vi "MiPS_set.vi"(5 "Target Current":dbl, 6 "stop":bool, 7 "Ramp Rate (A/min)":dbl, 8 "error in":errorcluster, 9 "ISOBUS address":T5, 11 "ref_in":T1) -> (0 "error out":errorcluster, 1 "PSU Act Stat":T4, 3 "ref_out":T1, 4 "iPS_msg":string caption="Msg.")   [LabVIEW 2019]
uses:
  Mercury iXX Modules/Public/Controls/ISOBus Address.ctl
  Mercury iXX Modules/Public/Libraries/Magnet/Controls/PSU Actions.ctl
  Mercury iXX Modules/Public/Controls/Mercury Reference.ctl
  Mercury iXX Modules/Public/Controls/Comms Transport Layer.ctl
  Mercury iXX Modules/Private/Controls/Query Dynamic Reference.ctl
  Mercury iXX Modules/Public/Libraries/Magnet/Signals/Set/Target Current (Set).vi
  Mercury iXX Modules/Public/Libraries/Magnet/Signals/Set/Target Current Rate (Set).vi
  Mercury iXX Modules/Public/Libraries/Magnet/Configuration/Set/PSU Action Status (Set).vi
  Mercury iXX Modules/Public/Libraries/Magnet/Configuration/Read/PSU Action Status (Read).vi
  Mercury iXX Modules/Mercury iXX.lvlib
  Mercury iXX Modules/Public/Libraries/Magnet.lvlib
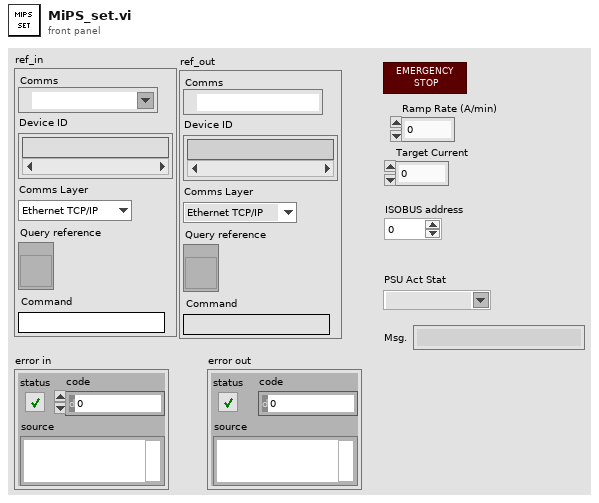
[diagram p1: front panel]
types:
  T1 = typedef "Mercury iXX.lvlib/Mercury Reference.ctl" = cluster{"Comms":refnum<visa-resource-name>, "Device ID":string[], "Comms Layer":T2, "Command":string, "Query reference":T3}
  T2 = typedef "Mercury iXX.lvlib/Comms Transport Layer.ctl" = enum16{"Ethernet TCP/IP", "USB", "ISOBus - RS-232", "GPIB"}
  T3 = typedef "Mercury iXX.lvlib/Query Dynamic Reference.ctl" = refnum<vi>
  T4 = typedef "Mercury iXX.lvlib/Magnet.lvlib/PSU Actions.ctl" = string
  T5 = typedef "Mercury iXX.lvlib/ISOBus Address.ctl" = i32
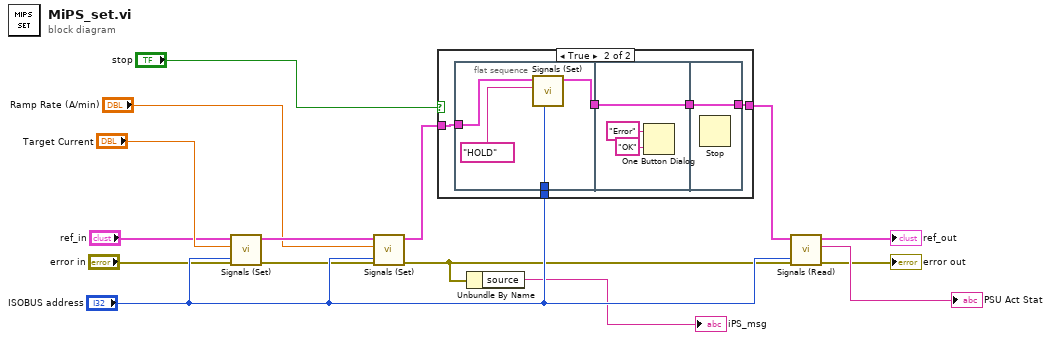
[diagram p0: block diagram]
diagram:
  n1 = call-poly "Signals (Set).vi"("ISOBUS address"="ISOBUS address", "error in"="error in", "Target Current"="Target Current", "Mercury Reference In"="ref_in") -> ("error out"=w4:errorcluster, "Mercury Reference Out"=w3:T1)  [unwired: 4 in, 2 out]
  n2 = call-poly "Signals (Set).vi"("ISOBUS address"="ISOBUS address", "error in"=w4, "Target Current Rate"="Ramp Rate (A/min)", "Mercury Reference In"=w3) -> ("error out"=w13:errorcluster, "Mercury Reference Out"=w6:T1)  [unwired: 4 in, 2 out]
  n3 = case shown="True" "stop" {
    tunnel: w6 -> [w16 w21]
    tunnel: [w16 w20] -> w7
    tunnel: "ISOBUS address" -> [_ w17]
    frame False {
    }
    frame True {
      n4 = flat-sequence {
        tunnel: w21 -> [w24]
        tunnel: [w23] -> w19
        tunnel: w17 -> [w22]
        tunnel: w19 -> [w28]
        tunnel: [w28] -> w18
        tunnel: [w29] -> w20
        tunnel: w18 -> [w29]
        frame #0 {
          n5 = call-poly "Signals (Set).vi"("ISOBUS address"=w22, "PSU Act Stat"=T4 "HOLD", "Mercury Reference In"=w24) -> ("Mercury Reference Out"=w23:T1)  [unwired: 5 in, 3 out]
        }
        frame #1 {
          n6 = One Button Dialog(message="Error", button name ("OK")="OK") -> ()  [unwired: 1 out]
        }
        frame #2 {
          n7 = Stop() -> ()  [unwired: 1 in]
        }
      }
    }
  }
  n8 = Unbundle By Name(w13) -> ("source"=→"iPS_msg":string)
  n9 = call-poly "Signals (Read).vi"("ISOBUS address"="ISOBUS address", "error in"=w13, "Mercury Reference In"=w7) -> ("error out"=→"error out":errorcluster, "PSU Act Stat"=→"PSU Act Stat":T4, "Mercury Reference Out"=→"ref_out":T1)  [unwired: 5 in, 1 out]
